vi "Size.vi"(8 "error in (no error)":errorcluster, 11 "Abs_Waveform in":refnum<class "Abs_Waveform.lvclass">) -> (0 "error out":errorcluster, 2 "size":i32, 3 "Abs_Waveform out":refnum<class "Abs_Waveform.lvclass">)   [LabVIEW 2021, in "Abs_Waveform.lvclass"]
uses:
  Abs_Waveform.lvclass
  Abs_Waveform.lvclass/Abs_Waveform.ctl
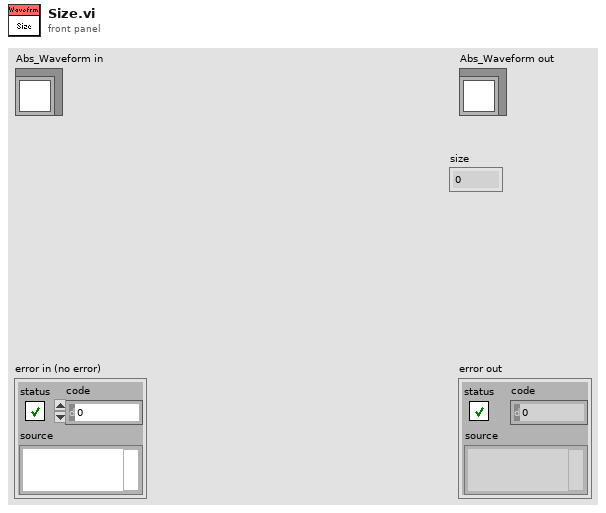
[diagram p1: front panel]
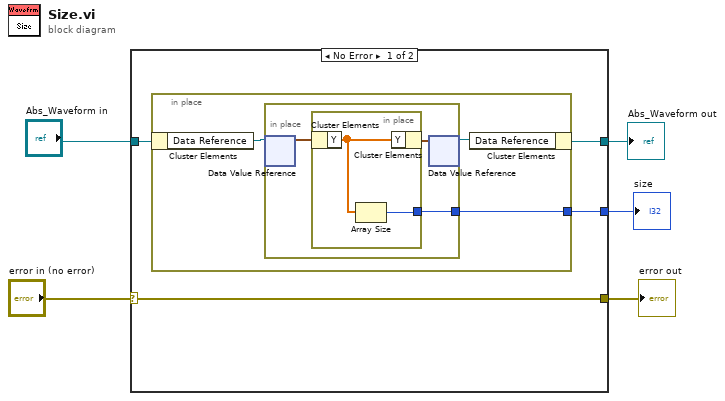
[diagram p0: block diagram]
diagram:
  n1 = case shown="No Error" "error in (no error)" {
    selector: "error in (no error)" -> [w6 w18]
    tunnel: [w9 w19] -> w5
    tunnel: "Abs_Waveform in" -> [w8 w19]
    tunnel: [w7 _] -> w3
    tunnel: [w6 w18] -> w1
    frame No Error {
      n2 = in-place {
        in-place-border: [w10] -> w7
        n3 = in-place-cluster #1(w8) -> ("Data Reference"=w12:refnum<data-value>)
        n4 = in-place {
          in-place-border: [w13] -> w10
          n5 = in-place-dvr #2(w12) -> (w15:waveform(dbl))  [unwired: 1 out]
          n6 = in-place {
            in-place-border: [w16] -> w13
            n7 = in-place-cluster #3(w15) -> ("Y"=w17:dbl[])
            n8 = Array Size(array=w17) -> (size(s)=w16:i32)
            n9 = in-place-cluster #3("Y"=w17) -> (w14:waveform(dbl))
          }
          n10 = in-place-dvr #2(w14) -> (w11:refnum<data-value>)  [unwired: 1 out]
        }
        n11 = in-place-cluster #1("Data Reference"=w11) -> (w9:refnum<class "Abs_Waveform.lvclass">)
      }
    }
    frame Error {
    }
  }
  "error out" <- w1
  "Abs_Waveform out" <- w5
  "size" <- w3
